vi "citTemplate.queueRepository.vi"(0 "mode (get queue handle)":T1=enum."get queue handle(s)", 1 "queue in":refnum<queue>, 2 "instance (0)":i32, 7 "event in":variant, 9 "(flatten) data in":string, 11 "error in (no error)":errorcluster) -> (3 "queue out":refnum<queue>, 4 "queueHandle(s) out":refnum<queue>[](array[refnum]), 8 "eventIndex(s)":u32[](array[numeric]), 15 "error out":errorcluster)   [LabVIEW 2016]
uses:
  citTemplate.eventQueue.ctl
  citTemplate.queueData.ctl
  citTemplate.notifierHandle.ctl
  citTemplate.notifierData.ctl
  citTemplate.ackNotifier.ctl
  citTemplate.ackData.ctl
panel:
  out "error out 2":errorcluster
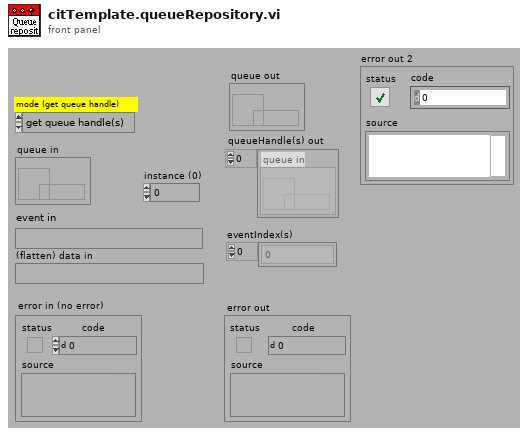
[diagram p1: front panel]
types:
  T1 = typedef "citTemplate.eventQueue.ctl" = enum16{"create queue", "get queue handle(s)", "destroy queue"}
  T2 = typedef "citTemplate.queueData.ctl" = cluster{"event index":u32, "(flatten) data in":string, "notifierHandle":T3}
  T3 = typedef "citTemplate.notifierHandle.ctl" = refnum<notifier>
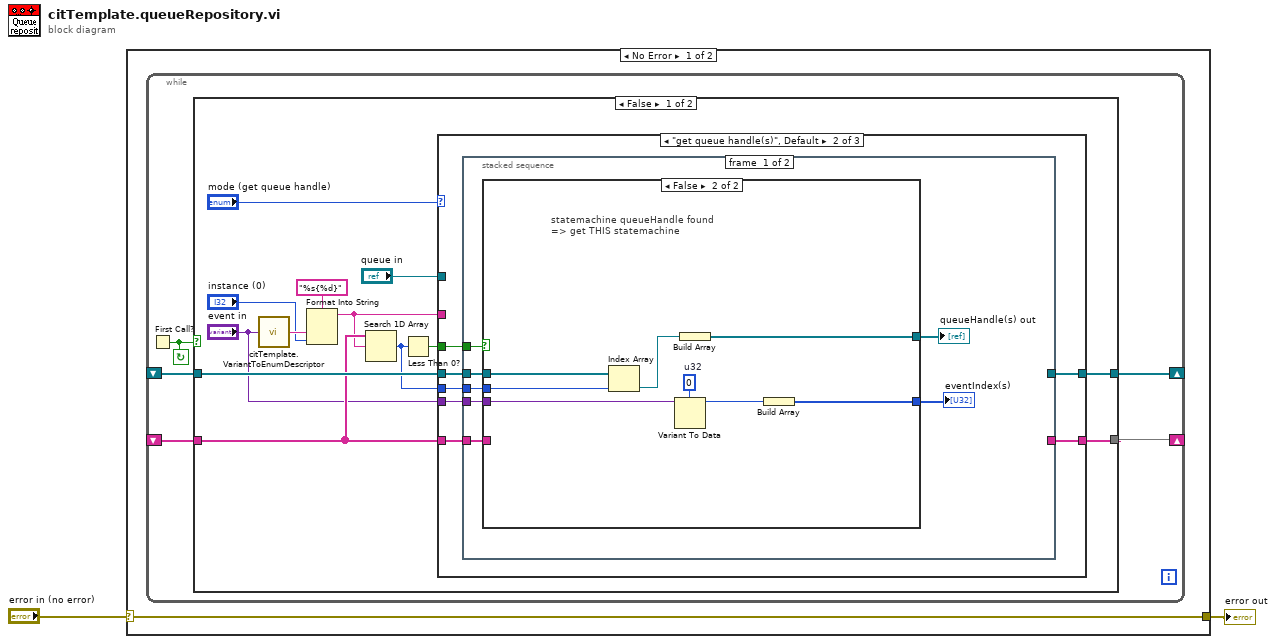
[diagram p0: block diagram]
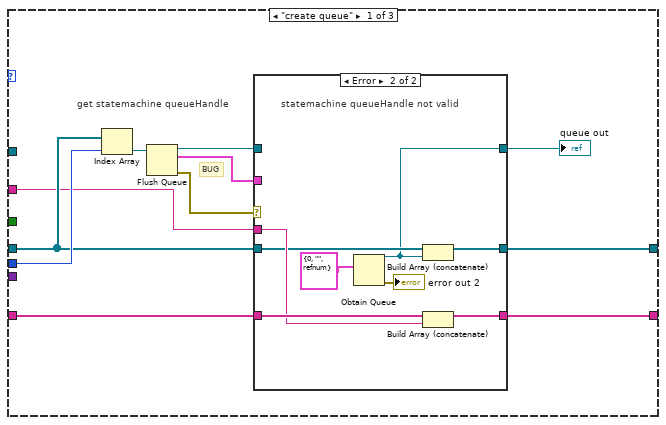
[diagram p2: hidden frame]
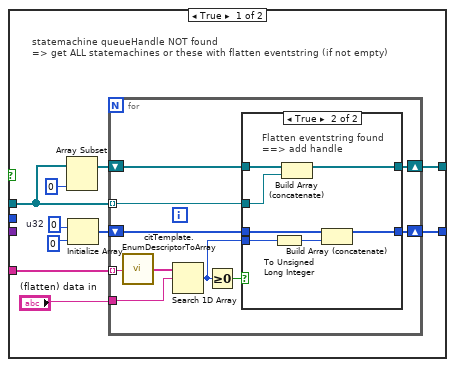
[diagram p4: hidden frame]
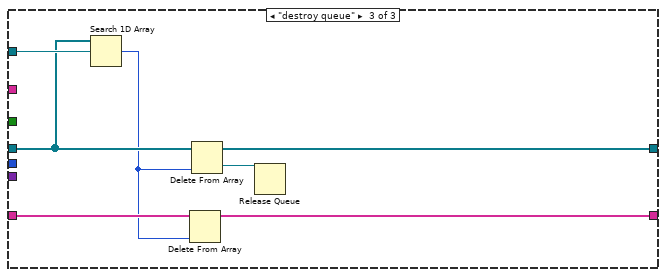
[diagram p7: hidden frame]
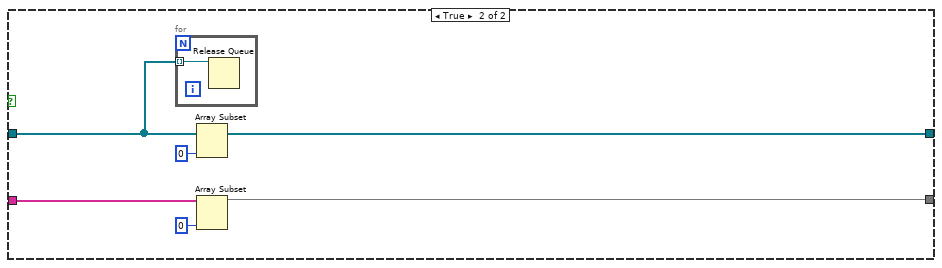
[diagram p8: hidden frame]
diagram:
  n1 = case shown="No Error" "error in (no error)" {
    selector: "error in (no error)" -> [w3 w111]
    tunnel: [w3 w111] -> w1
    frame No Error {
      n2 = while {
        shift-right: [w8] -> _
        shift-left: _ -> [w5]
        shift-right: [w7] -> _
        shift-left: _ -> [w6]
        stop <- w4 continue-if-true
        n3 = First Call?() -> (First Call?: T/F=w4:bool)
        n4 = case shown="False" w4 {
          tunnel: [w21 w105] -> w8
          tunnel: [w20 w106] -> w7
          tunnel: w6 -> [w19 w104]
          tunnel: w5 -> [w15 w107]
          frame False {
            n5 = call "citTemplate.VariantToEnumDescriptor.vi"("Variant enum data"="event in") -> ("enum type descriptor"=w12:string)  [unwired: 14 out]
            n6 = Format Into String(format string="%s{%d}", w12, "instance (0)") -> (resulting string=w10:string)  [unwired: 2 in, 1 out]
            n7 = Search 1D Array(1D array=w15, element=w10) -> (index of element=w16:i32)  [unwired: 1 out]
            n8 = Less Than 0?(x=w16) -> (x < 0?=w17:bool)
            n9 = case shown="\"get queue handle(s)\", Default" "mode (get queue handle)" {
              tunnel: [w26 w50 w99] -> w21
              tunnel: [w28 w49 w98] -> w20
              tunnel: w19 -> [w29 w48 w102]
              tunnel: w15 -> [w27 w47 w101]
              tunnel: w10 -> [w23 _ _]
              tunnel: w17 -> [_ w45 _]
              tunnel: w16 -> [w32 w46 _]
              tunnel: "queue in" -> [_ _ w103]
              tunnel: "event in" -> [_ w44 _]
              frame "create queue" {
                # "BUG"
                # "get statemachine queueHandle"
                n10 = Index Array(array=w29, index=w32) -> (element=w31:refnum<queue>)
                n11 = Flush Queue(queue=w31) -> (queue out=w30:refnum<queue>, remaining elements=w24:T2[], error out=w25:errorcluster)  [unwired: 1 in]
                n12 = case shown="Error" w25 {
                  tunnel: w27 -> [w35 w43]
                  tunnel: w23 -> [_ w42]
                  tunnel: w29 -> [w34 w41]
                  tunnel: [w34 w40] -> w28
                  tunnel: [w35 w39] -> w26
                  tunnel: [w33 w38] -> w22
                  tunnel: w30 -> [w33 _]
                  tunnel: w24 -> [_ _]
                  frame No Error {
                    # "statemachine queueHandle valid"
                  }
                  frame Error {
                    # "statemachine queueHandle not valid"
                    n13 = Obtain Queue(element data type=T2 {"event index"=0, "(flatten) data in"="", "notifierHandle"=refnum} ("queueData")) -> (queue out=w38:refnum<queue>, error out=→"error out 2":errorcluster)  [unwired: 3 in, 2 out]
                    n14 = Build Array (concatenate)(w41, w38) -> (w40:refnum<queue>[])
                    n15 = Build Array (concatenate)(w43, w42) -> (w39:string[])
                  }
                }
                "queue out" <- w22
              }
              frame "get queue handle(s)", Default {
                n16 = stacked-sequence {
                  tunnel: w47 -> [w54 w95]
                  tunnel: [_ w96] -> w49
                  tunnel: w48 -> [w57 w96]
                  tunnel: [_ w95] -> w50
                  tunnel: w46 -> [w56 _]
                  tunnel: w45 -> [w55 _]
                  tunnel: w44 -> [w51 _]
                  frame #0 {
                    n17 = case shown="False" w55 {
                      tunnel: w57 -> [w66 w94]
                      tunnel: w56 -> [_ w92]
                      tunnel: w54 -> [w67 _]
                      tunnel: [w59 w90] -> w53
                      tunnel: [w58 w91] -> w52
                      tunnel: w51 -> [_ w87]
                      frame True {
                        w61 = u32 0  # u32
                        # "statemachine queueHandle NOT found\n=> get ALL statemachines or these with flatten eventstring (if not empty)"
                        n18 = Array Subset(array=w66, length=0) -> (w64:refnum<queue>[])  [unwired: 1 in]
                        n19 = Initialize Array(w61, 0 ("length")) -> (w62:u32[])
                        n20 = for {
                          tunnel: w66 -> [w77] mode=indexing
                          tunnel: w67 -> [w76] mode=indexing
                          tunnel: "(flatten) data in" -> [w74]
                          shift-right: [w71] -> w59
                          shift-left: w64 -> [w72]
                          shift-right: [w68] -> w58
                          shift-left: w62 -> [w70]
                          n21 = call "citTemplate.EnumDescriptorToArray.vi"("enum type descriptor"=w76) -> ("array"=w75:string[])  [unwired: 14 out]
                          n22 = Search 1D Array(1D array=w75, element=w74) -> (index of element=w69:i32)  [unwired: 1 out]
                          n23 = Greater Or Equal To 0?(x=w69) -> (x >= 0?=w73:bool)
                          n24 = case shown="True" w73 {
                            tunnel: w77 -> [_ w85]
                            tunnel: w72 -> [w79 w86]
                            tunnel: [w79 w84] -> w71
                            tunnel: w70 -> [w78 w81]
                            tunnel: w69 -> [_ w83]
                            tunnel: [w78 w80] -> w68
                            frame False {
                              # "Flatten eventstring not found"
                            }
                            frame True {
                              # "Flatten eventstring found\n==> add handle"
                              n25 = To Unsigned Long Integer(number=w83) -> (unsigned 32bit integer=w82:u32)
                              n26 = Build Array (concatenate)(w86, w85) -> (w84:refnum<queue>[])
                              n27 = Build Array (concatenate)(w81, w82) -> (w80:u32[])
                            }
                          }
                        }
                      }
                      frame False {
                        w89 = u32 0  # u32
                        # "statemachine queueHandle found\n=> get THIS statemachine"
                        n28 = Index Array(array=w94, index=w92) -> (element=w93:refnum<queue>)
                        n29 = Variant To Data(type=w89, Variant=w87) -> (data=w88:u32)  [unwired: 1 in, 1 out]
                        n30 = Build Array(w93) -> (w90:refnum<queue>[])
                        n31 = Build Array(w88) -> (w91:u32[])
                      }
                    }
                    "queueHandle(s) out" <- w53
                    "eventIndex(s)" <- w52
                  }
                  frame #1 {
                    # "datatunnel"
                  }
                }
              }
              frame "destroy queue" {
                n32 = Search 1D Array(1D array=w102, element=w103) -> (index of element=w100:i32)  [unwired: 1 out]
                n33 = Delete From Array(array=w101, index=w100) -> (array with subset deleted=w99:string[])  [unwired: 1 in, 1 out]
                n34 = Delete From Array(array=w102, index=w100) -> (deleted portion=w97:refnum<queue>, array with subset deleted=w98:refnum<queue>[])  [unwired: 1 in]
                n35 = Release Queue(queue=w97) -> ()  [unwired: 1 in, 4 out]
              }
            }
          }
          frame True {
            n36 = for {
              tunnel: w104 -> [w110] mode=indexing
              n37 = Release Queue(queue=w110) -> ()  [unwired: 1 in, 4 out]
            }
            n38 = Array Subset(array=w104, length=0) -> (w106:refnum<queue>[])  [unwired: 1 in]
            n39 = Array Subset(array=w107, length=0) -> (w105:string[])  [unwired: 1 in]
          }
        }
      }
    }
    frame Error {
    }
  }
  "error out" <- w1
